vi "array_sorting_without_internal_function.vi"() -> ()   [LabVIEW 2019]
panel:
  in  "?":bool
  in  "input_array":string[](array[string])
  out "given_array":string[](array[string])
  out "sorted":string[](array[string])
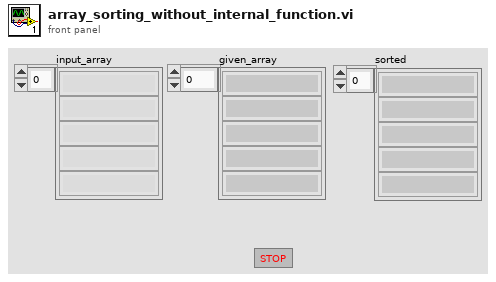
[diagram p1: front panel]
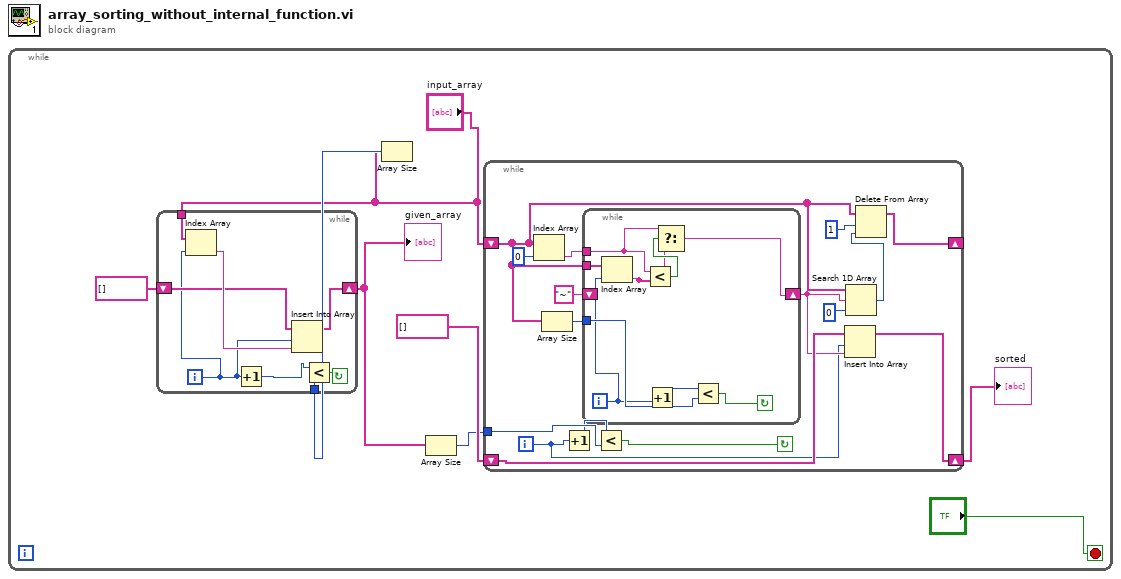
[diagram p0: block diagram]
diagram:
  n1 = while {
    stop <- "?" stop-if-true
    n2 = Array Size(array="input_array") -> (size(s)=w4:i32)
    n3 = while {
      tunnel: "input_array" -> [w16]
      shift-right: [w13] -> w3
      shift-left: string[] [] -> [w14]
      tunnel: w4 -> [w12]
      i -> [w9]
      stop <- w11 continue-if-true
      n4 = Index Array(array=w16, index=w9) -> (element=w15:string)
      n5 = Increment(x=w9) -> (x+1=w10:i32)
      n6 = Insert Into Array(array=w14, index=w9, new element=w15) -> (w13:string[])
      n7 = Less?(x=w10, y=w12) -> (x < y?=w11:bool)
    }
    "given_array" <- w3
    n8 = Array Size(array=w3) -> (size(s)=w5:i32)
    n9 = while {
      shift-right: [w29] -> _
      shift-left: "input_array" -> [w25]
      shift-right: [w27] -> w7
      shift-left: string[] [] -> [w28]
      tunnel: w5 -> [w26]
      i -> [w19]
      stop <- w32 continue-if-true
      n10 = Index Array(array=w25, index=0) -> (element=w23:string)
      n11 = Array Size(array=w25) -> (size(s)=w24:i32)
      n12 = Increment(x=w19) -> (x+1=w18:i32)
      n13 = while {
        tunnel: w25 -> [w41]
        tunnel: w24 -> [w39]
        tunnel: w23 -> [w36]
        shift-right: [w34] -> w22
        shift-left: "~" ("String") -> [_]
        i -> [w33]
        stop <- w40 continue-if-true
        n14 = Index Array(array=w41, index=w33) -> (element=w35:string)
        n15 = Less?(x=w36, y=w35) -> (x < y?=w37:bool)
        n16 = Increment(x=w33) -> (x+1=w38:i32)
        n17 = Select(t=w36, s=w37, f=w35) -> (s? t:f=w34:string)
        n18 = Less?(x=w38, y=w39) -> (x < y?=w40:bool)
      }
      n19 = Less?(x=w18, y=w26) -> (x < y?=w32:bool)
      n20 = Insert Into Array(array=w28, index=w19, new element=w22) -> (w27:string[])
      n21 = Search 1D Array(1D array=w25, element=w22, start index (0)=0) -> (index of element=w21:i32)
      n22 = Delete From Array(array=w25, length=1, index=w21) -> (array with subset deleted=w29:string[])  [unwired: 1 out]
    }
    "sorted" <- w7
  }
